vi "KeySight 53230A VISA Test.vi"() -> ()   [LabVIEW 2018]
uses:
  <instrlib>/Agilent 532XX Series/Public/Configure/Configure Channel (Basic).vi
  <instrlib>/Agilent 532XX Series/Public/Configure/Configure Channel (Voltage Range).vi
  <instrlib>/Agilent 532XX Series/Public/Configure/Configure Channel (Threshold Voltage).vi
  <instrlib>/Agilent 532XX Series/Public/Configure/Configure Channel (Slop).vi
  <instrlib>/Agilent 532XX Series/Public/Configure/Measurement/Configure Measurement (Totalize Timed).vi
  <instrlib>/Agilent 532XX Series/Public/Data/Read Measurement (Single).vi
  <instrlib>/Agilent 532XX Series/Agilent 532XX Series.lvlib
panel:
  out "Numeric":i32
  out "Measurement":dbl format="%#_12g"
  in  "stop":bool
  out "error out":errorcluster
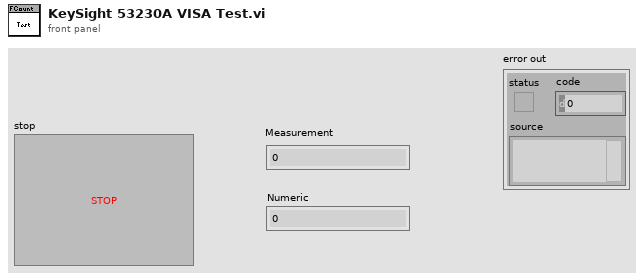
[diagram p1: front panel]
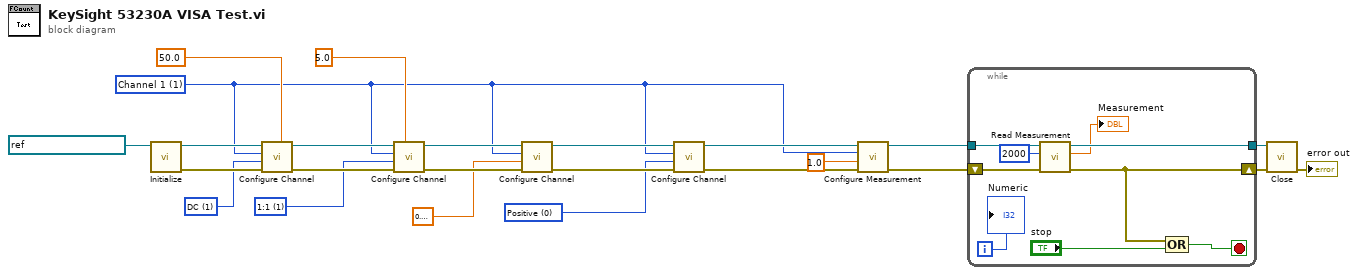
[diagram p0: block diagram]
diagram:
  w7 = 0 items=["Positive", "Negative"] ("Active Edge (1: Negative)")
  w14 = 1 items=["1:1"=1, "10:1"=10] ("Probe Factor ( 1:1)")
  w17 = 50.0 items=["50"=50.0, "1E+6"=1000000.0] ("Impedance (1E+6 Ohm)")
  w18 = 1 items=["AC", "DC"] ("Coupling (0: AC)")
  w2 = 1 items=["Channel 1"=1, "Channel 2"=2] ("Channel (1: Channel 1)")
  n1 = call <instrlib>:"Initialize.vi"("VISA resource name"=refnum<visa-resource-name> "KeySight_53230A") -> ("error out"=w21:errorcluster, "VISA resource name out"=w22:refnum<visa-resource-name>)  [unwired: 9 in]
  n2 = call-poly <instrlib>:"Configure Channel.vi"("Impedance (1E+6 Ohm)"=w17, "error in (no error)"=w21, "Coupling (0: AC)"=w18, "Channel (1: Channel 1)"=w2, "VISA resource name"=w22) -> ("error out"=w16:errorcluster, "VISA resource name out"=w15:refnum<visa-resource-name>)  [unwired: 5 in]
  n3 = call-poly <instrlib>:"Configure Channel.vi"("Voltage Range (5V)"=5.0, "error in (no error)"=w16, "Probe Factor ( 1:1)"=w14, "Channel (1: Channel 1)"=w2, "VISA resource name"=w15) -> ("error out"=w12:errorcluster, "VISA resource name out"=w10:refnum<visa-resource-name>)  [unwired: 5 in]
  n4 = call-poly <instrlib>:"Configure Channel.vi"("error in (no error)"=w12, "Threshold Voltage (0 V)"=0.30000000000000004, "Channel (1: Channel 1)"=w2, "VISA resource name"=w10) -> ("error out"=w8:errorcluster, "VISA resource name out"=w9:refnum<visa-resource-name>)  [unwired: 6 in]
  n5 = call-poly <instrlib>:"Configure Channel.vi"("error in (no error)"=w8, "Active Edge (1: Negative)"=w7, "Channel (1: Channel 1)"=w2, "VISA resource name"=w9) -> ("error out"=w4:errorcluster, "VISA resource name out"=w3:refnum<visa-resource-name>)  [unwired: 6 in]
  n6 = call-poly <instrlib>:"Configure Measurement.vi"("error in (no error)"=w4, "Timed Totalize (0.1 s)"=1.0, "Channel (1: Channel 1)"=w2, "VISA resource name"=w3) -> ("error out"=w5:errorcluster, "VISA resource name out"=w6:refnum<visa-resource-name>)  [unwired: 6 in]
  n7 = while {
    tunnel: w6 -> [w30]
    tunnel: [w29] -> w20
    shift-right: [w28] -> w19
    shift-left: w5 -> [w33]
    i -> [w25]
    stop <- w31 stop-if-true
    n8 = call-poly <instrlib>:"Read Measurement.vi"("error in (no error)"=w33, "Timeout (10000 ms)"=u32 2000, "VISA resource name"=w30) -> ("error out"=w28:errorcluster, "Measurement"=→"Measurement":dbl, "VISA resource name out"=w29:refnum<visa-resource-name>)  [unwired: 6 in]
    n9 = Compound Arithmetic op=OR(w28, "stop") -> (w31:bool)
    "Numeric" <- w25
  }
  n10 = call <instrlib>:"Close.vi"("error in (no error)"=w19, "VISA resource name"=w20) -> ("error out"=→"error out":errorcluster)  [unwired: 9 in]
